vi "RecyclingContainerFromRight.vi"(0 "Boolean In":bool) -> (7 "Boolean Out":bool)   [LabVIEW 2014]
uses:
  Support Files/RC PickupStates.ctl
  Support Files/Global Data!!!.vi
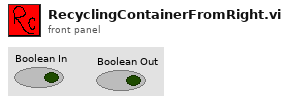
[diagram p1: front panel]
types:
  T1 = typedef "RC PickupStates.ctl" = enum16{"PickToteUp", "Disengage", "Drop", "Hold", "Lift", "Engage1Stage", "Rest", "DropAgain", "Done", "Lift.5", "Pause4Jones"}
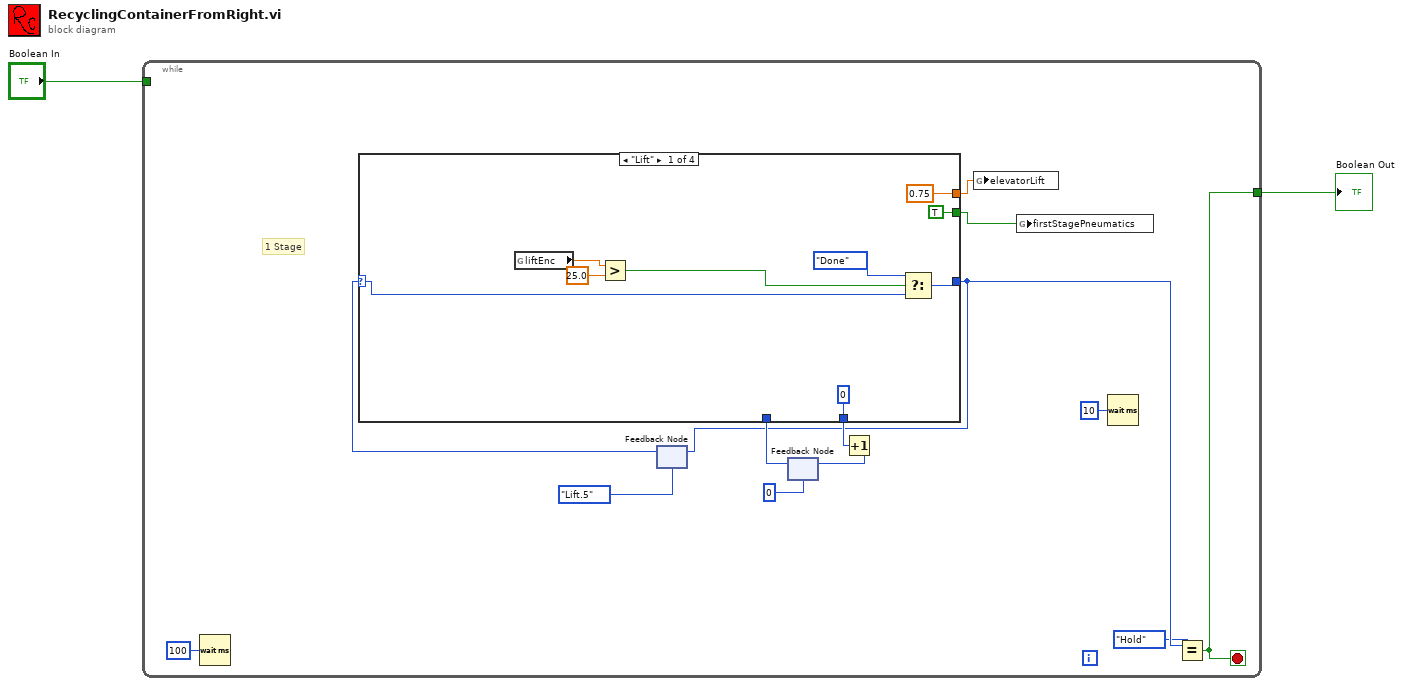
[diagram p0: block diagram]
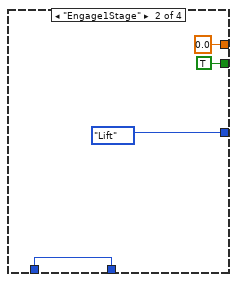
[diagram p2: hidden frame]
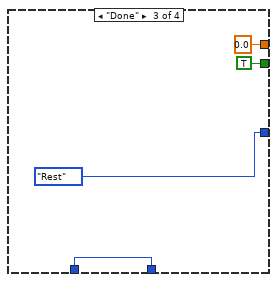
[diagram p3: hidden frame]
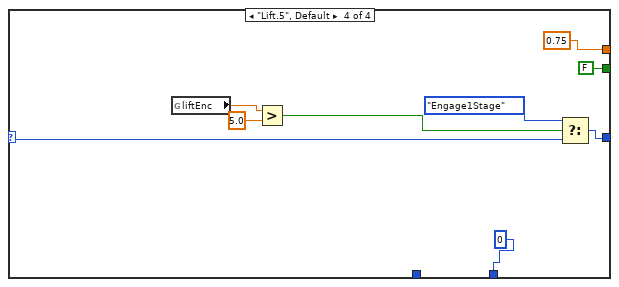
[diagram p4: hidden frame]
diagram:
  n1 = while {
    tunnel: "Boolean In" -> [_]
    tunnel: [w6] -> w1
    stop <- w6 stop-if-true
    # "1 Stage"
    n2 = Wait (ms)(milliseconds to wait=u32 100) -> ()  [unwired: 1 out]
    n3 = feedback #1(RC_PickupStates."Lift.5") -> (w13:T1)
    n4 = feedback #2(0 ("t")) -> (w11:i32)
    n5 = case shown="\"Lift\"" w13 {
      selector: w13 -> [w22 _ _ w36]
      tunnel: [w23 RC_PickupStates."Lift" ("t") RC_PickupStates."Rest" w37] -> w8
      tunnel: w11 -> [_ w28 w32 _]
      tunnel: [0 ("t") w28 w32 0 ("t")] -> w10
      tunnel: [0.75 0.0 0.0 0.75] -> w5
      tunnel: [TRUE TRUE TRUE FALSE] -> w4
      frame "Lift" {
        n6 = global read "Global Data!!!.vi" "liftEnc"() -> (w20:dbl)
        n7 = Greater?(x=w20, y=25.0) -> (0:w18:bool)
        n8 = Select(t=RC_PickupStates."Done", s=w18, f=w22) -> (s? t:f=w23:T1)
      }
      frame "Engage1Stage" {
      }
      frame "Done" {
      }
      frame "Lift.5", Default {
        n9 = global read "Global Data!!!.vi" "liftEnc"() -> (w40:dbl)
        n10 = Greater?(x=w40, y=5.0) -> (0:w38:bool)
        n11 = Select(t=RC_PickupStates."Engage1Stage", s=w38, f=w36) -> (s? t:f=w37:T1)
      }
    }
    n12 = feedback-in #1(w8) -> ()
    n13 = Increment(x=w10) -> (x+1=w9:i32)
    n14 = feedback-in #2(w9) -> ()
    n15 = global write "Global Data!!!.vi" "elevatorLift"(w5) -> ()
    n16 = global write "Global Data!!!.vi" "firstStagePneumatics"(w4) -> ()
    n17 = Wait (ms)(milliseconds to wait=u32 10) -> ()  [unwired: 1 out]
    n18 = Equal?(x=w8, y=RC_PickupStates."Hold") -> (x = y?=w6:bool)
  }
  "Boolean Out" <- w1
